vi "Test Invalid Write - Flush Error.vi"() -> ()   [LabVIEW 2024]
uses:
  Sift API/Sift Client.lvclass
  Sift Client.lvlib
  Mock Sift Proxy Server/Mock Sift Proxy Server.lvclass
  Sift API/Types/Data Type.ctl
panel:
  out "Server Error":errorcluster
  out "Success 2":bool
  out "Error 2":errorcluster
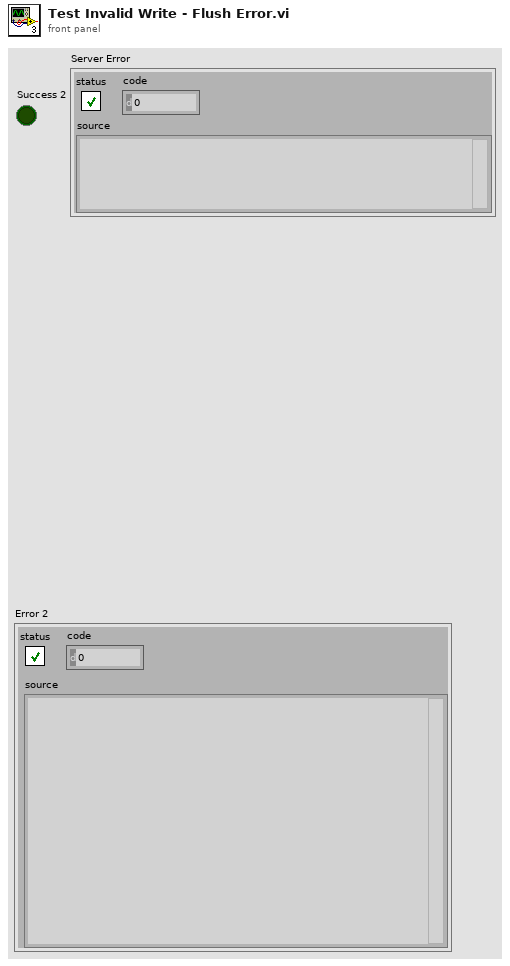
[diagram p1: front panel]
types:
  T1 = typedef "Sift Client.lvlib/Data Type.ctl" = enum8{"double", "float", "uint64", "int64", "uint32", "int32", "bool", "bit field", "enum", "string"}
  T2 = typedef "Sift Client.lvlib/JSON Response.ctl" = cluster{"status":bool, "data":variant}
  T3 = typedef "Sift Client.lvlib/Channel Config.ctl" = cluster{"name":string, "data_type":T1, "description":string, "component":string, "unit":string, "bit_field_elements":T4[], "enum_types":T5[]}
  T4 = typedef "Sift Client.lvlib/Bit Field.ctl" = cluster{"index":u32, "bit_count":u32, "name":string}
  T5 = typedef "Sift Client.lvlib/Enum.ctl" = cluster{"Key":u32, "Name":string}
  T6 = typedef "Sift Client.lvlib/Timestamp.ctl" = cluster{"seconds":i64, "nanos":i32}
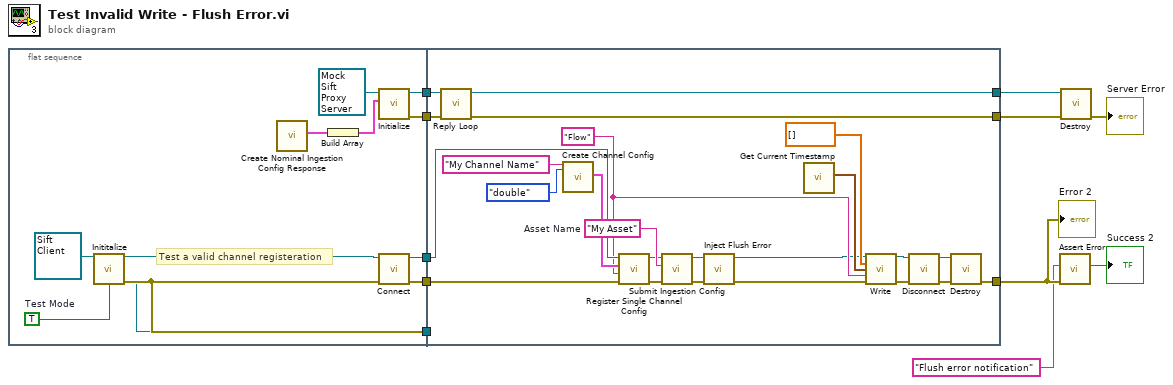
[diagram p0: block diagram]
diagram:
  n1 = flat-sequence {
    tunnel: [w22] -> w12
    tunnel: [w19] -> w11
    tunnel: [w18] -> w10
    tunnel: [w17] -> w9
    tunnel: [w16] -> w8
    tunnel: [w15] -> w7
    tunnel: [w39] -> w6
    tunnel: w12 -> [w40]
    tunnel: [w46] -> w2
    tunnel: w11 -> [_]
    tunnel: w10 -> [_]
    tunnel: w9 -> [w38]
    tunnel: w8 -> [w37]
    tunnel: w7 -> [w34]
    tunnel: [w33] -> w5
    frame #0 {
      w20 = TRUE  # Test Mode
      # "Test a valid channel registeration"
      n2 = call-dynamic "Inititalize.vi"("Sift Client in"=refnum<class "Sift Client.lvclass"> refnum ("Sift Client.lvlib:Sift Client.lvclass"), "Test Mode"=w20) -> ("Sift Client out"=w18:refnum<class "Sift Client.lvclass">, "error out"=w19:errorcluster)  [unwired: 12 in]
      n3 = call "Create Nominal Ingestion Config Response.vi"() -> ("output cluster"=w14:T2)  [unwired: 11 in]
      n4 = Build Array(w14) -> (w13:T2[])
      n5 = call-dynamic "Initialize.vi"("Mock Replies"=w13, "Mock Sift Proxy Server in"=refnum<class "Mock Sift Proxy Server.lvclass"> refnum ("Mock Sift Proxy Server.lvclass")) -> ("error out"=w15:errorcluster, "Mock Sift Proxy Server out"=w22:refnum<class "Mock Sift Proxy Server.lvclass">)  [unwired: 8 in]
      n6 = call-dynamic "Connect.vi"("error in (no error)"=w19, "Sift Client in"=w18) -> ("error out"=w17:errorcluster, "Sift Client out"=w16:refnum<class "Sift Client.lvclass">)  [unwired: 7 in, 1 out]
    }
    frame #1 {
      w42 = "My Asset"  # Asset Name
      w28 = "Flow" ("Flow Name")
      n7 = call-dynamic "Reply Loop.vi"("error in (no error)"=w34, "Mock Sift Proxy Server in"=w40) -> ("error out"=w33:errorcluster, "Mock Sift Proxy Server out"=w39:refnum<class "Mock Sift Proxy Server.lvclass">)  [unwired: 8 in]
      n8 = call "Create Channel Config.vi"("Name"="My Channel Name", "Data Type"=Data_Type."double" ("Enum")) -> ("Output"=w43:T3)  [unwired: 17 in]
      n9 = call-dynamic "Register Single Channel Config.vi"("error in (no error)"=w38, "Flow Name"=w28, "Channel Config"=w43, "Sift Client in"=w37) -> ("error out"=w47:errorcluster, "Sift Client out"=w41:refnum<class "Sift Client.lvclass">)  [unwired: 6 in]
      n10 = call-dynamic "Submit Ingestion Config.vi"("error in (no error)"=w47, "Asset Name"=w42, "Sift Client in"=w41) -> ("error out"=w31:errorcluster, "Sift Client out"=w32:refnum<class "Sift Client.lvclass">)  [unwired: 6 in, 1 out]
      n11 = call-dynamic "Inject Flush Error.vi"("error in (no error)"=w31, "Sift Client in"=w32) -> ("error out"=w26:errorcluster, "Sift Client out"=w27:refnum<class "Sift Client.lvclass">)  [unwired: 8 in]
      n12 = call "Get Current Timestamp.vi"() -> ("Timestamp"=w30:T6)  [unwired: 11 in]
      n13 = call-dynamic "Write.vi"("Sift Client in"=w27, "Values"=dbl[] [], "Timestamp"=w30, "Flow Name"=w28, "error in (no error)"=w26) -> ("Sift Client out"=w25:refnum<class "Sift Client.lvclass">, "error out"=w24:errorcluster)  [unwired: 9 in]
      n14 = call-dynamic "Disconnect.vi"("error in (no error)"=w24, "Sift Client in"=w25) -> ("error out"=w35:errorcluster, "Sift Client out"=w36:refnum<class "Sift Client.lvclass">)  [unwired: 8 in]
      n15 = call-dynamic "Destroy.vi"("error in (no error)"=w35, "Sift Client in"=w36) -> ("error out"=w46:errorcluster)  [unwired: 8 in, 1 out]
    }
  }
  n16 = call "Assert Error.vi"("Error"=w2, "Error String"="Flush error notification") -> ("Success"=→"Success 2":bool)  [unwired: 9 in]
  n17 = call-dynamic "Destroy.vi"("error in (no error)"=w5, "Mock Sift Proxy Server in"=w6) -> ("error out"=→"Server Error":errorcluster)  [unwired: 8 in, 1 out]
  "Error 2" <- w2
